vi "SendMessageToConsole.vi"(1 "Message String":string) -> ()   [LabVIEW 2019]
doc: "This VI sends a message to the driver station console whenever the message changes."
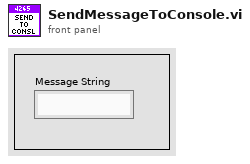
[diagram p1: front panel]
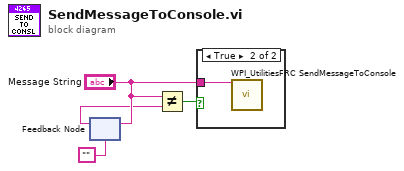
[diagram p0: block diagram]
diagram:
  n1 = feedback #1("") -> (w2:string)
  n2 = feedback-in #1("Message String") -> ()
  n3 = Not Equal?(x="Message String", y=w2) -> (x != y?=w1:bool)
  n4 = case shown="True" w1 {
    tunnel: "Message String" -> [_ w5]
    frame False {
    }
    frame True {
      n5 = call <vilib>:"WPI_UtilitiesFRC SendMessageToConsole.vi"("Message"=w5) -> ()  [unwired: 14 in, 1 out]
    }
  }
